vi "Get_data form SQL.vi"(8 "error in (no error)":errorcluster, 11 "Export":bool) -> (0 "error out":errorcluster, 3 "data":string[][](array[string]))   [LabVIEW 2020]
uses:
  <vilib>/addons/database/Connection.llb/DB Tools Open Connec (Path).vi
  <vilib>/addons/database/Connection.llb/Conn Execute.vi
  <vilib>/addons/database/Recordset.llb/Rec Fetch Recordset Data (R).vi
  <vilib>/addons/database/Recordset.llb/Rec Destroy - Connection.vi
  <vilib>/addons/database/_DB Variant To Data/Database Variant To Data.xnode
  <vilib>/addons/database/NI_Database_API.lvlib
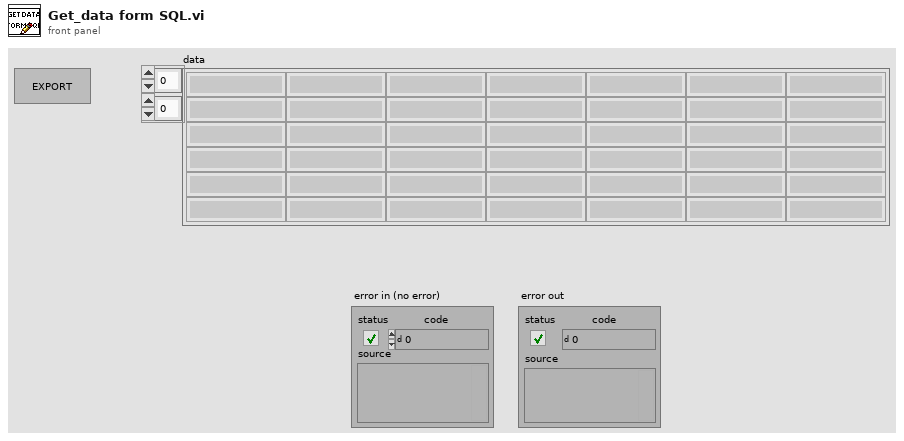
[diagram p1: front panel]
types:
  T1 = typedef "NI_Database_API.lvlib/Conn ObjectReference.ctl" = refnum<k1>
  T2 = typedef "NI_Database_API.lvlib/Rec ObjectReference.ctl" = refnum<k1>
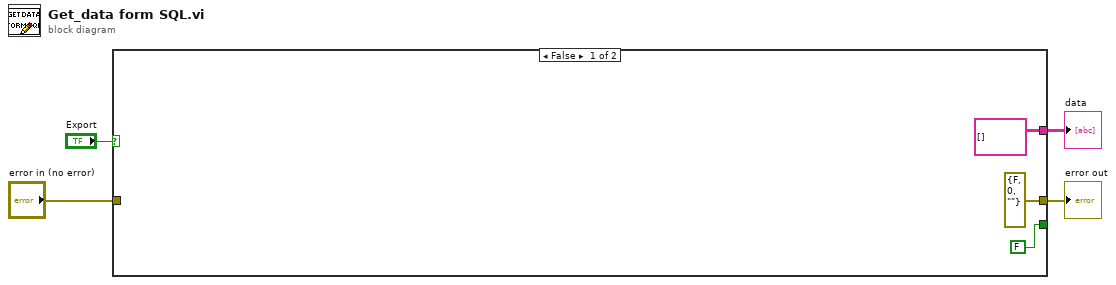
[diagram p0: block diagram]
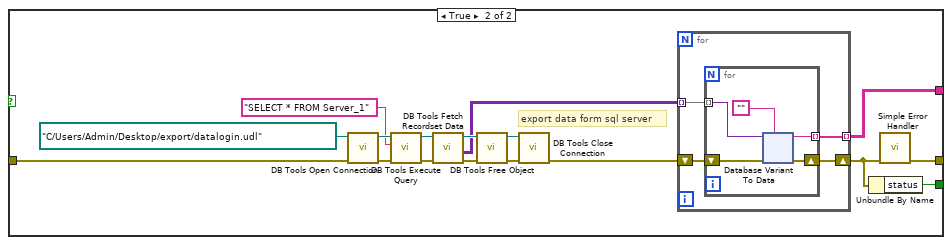
[diagram p2: hidden frame]
diagram:
  n1 = case shown="False" "Export" {
    tunnel: [errorcluster {"status"=FALSE, "code"=0, "source"=""} ("error out") w10] -> w4
    tunnel: [FALSE ("status") w14] -> _
    tunnel: "error in (no error)" -> [_ w9]
    tunnel: [string[][] [] w8] -> w1
    frame False {
    }
    frame True {
      # "export data form sql server"
      n2 = call-poly <vilib>:"DB Tools Open Connection.vi"("error in (no error)"=w9, "connection information"=path "C:/Users/Admin/Desktop/export/datalogin.udl" ("DB Handle")) -> ("error out"=w19:errorcluster, "connection reference"=w18:T1)  [unwired: 6 in]
      n3 = call-poly <vilib>:"DB Tools Execute Query.vi"("error in (no error)"=w19, "SQL query"="SELECT * FROM Server_1", "connection reference"=w18) -> ("error out"=w21:errorcluster, "recordset reference"=w22:T2)  [unwired: 5 in]
      n4 = call-poly <vilib>:"DB Tools Fetch Recordset Data.vi"("error in (no error)"=w21, "recordset reference"=w22) -> ("error out"=w20:errorcluster, "recordset data"=w13:variant[][], "recordset reference out"=w23:T2)  [unwired: 3 in]
      n5 = call-poly <vilib>:"DB Tools Free Object.vi"("error in (no error)"=w20, "recordset reference"=w23) -> ("error out"=w15:errorcluster, "connection reference"=w16:T1)  [unwired: 8 in]
      n6 = call <vilib>:"DB Tools Close Connection.vi"("error in (no error)"=w15, "connection reference"=w16) -> ("error out"=w12:errorcluster)  [unwired: 5 in]
      n7 = for {
        tunnel: w13 -> [w28] mode=indexing
        tunnel: [w27] -> w8 mode=indexing
        shift-right: [w25] -> w11
        shift-left: w12 -> [w26]
        n8 = for {
          tunnel: w28 -> [w33] mode=indexing
          tunnel: [w32] -> w27 mode=indexing
          shift-right: [w29] -> w25
          shift-left: w26 -> [w30]
          n9 = xnode "Database Variant To Data"("database variant"=w33, "error in (no error)"=w30, "type"="") -> ("data"=w32:string, "error out"=w29:errorcluster)
        }
      }
      n10 = Unbundle By Name(w11) -> ("status"=w14:bool)
      n11 = call <vilib>:"Simple Error Handler.vi"("error in (no error)"=w11) -> ("error out"=w10:errorcluster)  [unwired: 4 in, 4 out]
    }
  }
  "error out" <- w4
  "data" <- w1
